vi "WrapStrToFitButtonSize.vi"(0 "String in":string) -> (14 "Wrapped String":string)   [LabVIEW 2017, in "NEVSTOP QD Shortcuts.lvlib"]
uses:
  NEVSTOP QD Shortcuts.lvlib
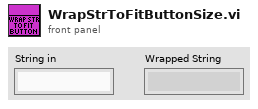
[diagram p1: front panel]
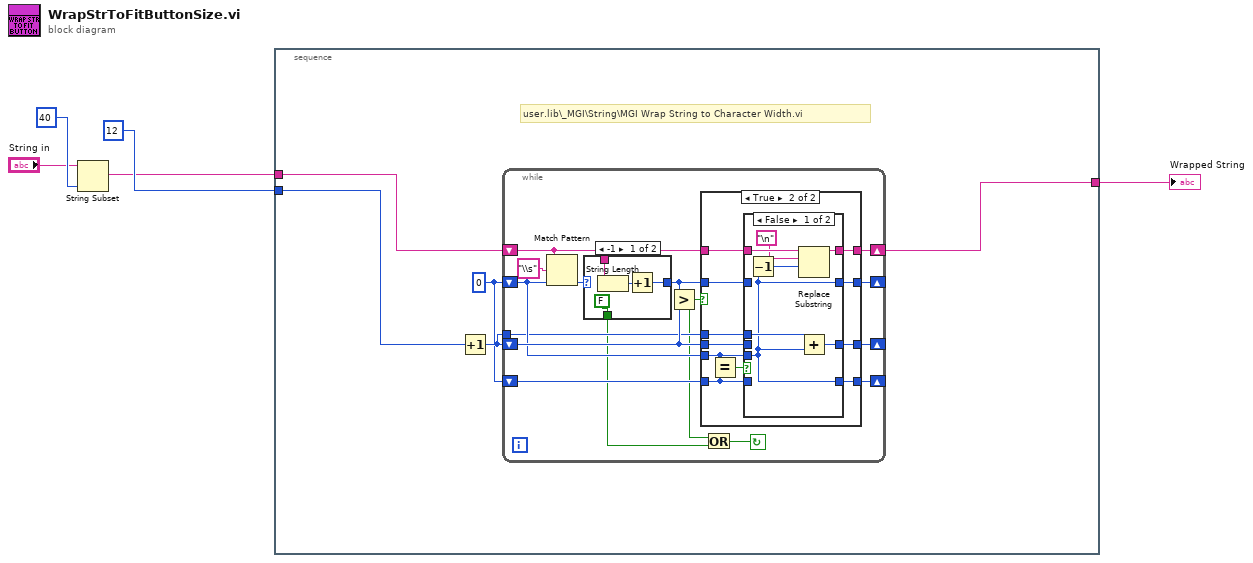
[diagram p0: block diagram]
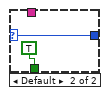
[diagram p2: hidden frame]
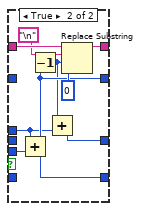
[diagram p4: hidden frame]
diagram:
  n1 = String Subset(string="String in", length (rest)=40 ("length (rest)")) -> (substring=w3:string)  [unwired: 1 in]
  n2 = stacked-sequence {
    tunnel: [w10] -> w2
    tunnel: 12 ("Wrap length(Characters)") -> [w9]
    tunnel: w3 -> [w6]
    frame #0 {
      w7 = 0
      # "user.lib\\_MGI\\String\\MGI Wrap String to Character Width.vi"
      n3 = Increment(x=w9) -> (x+1=w8:i32)
      n4 = while {
        shift-right: [w24] -> w10
        shift-left: w6 -> [w18]
        shift-right: [w23] -> _
        shift-left: w7 -> [w15]
        shift-right: [w21] -> _
        shift-left: w8 -> [w22]
        shift-right: [w16] -> _
        shift-left: w7 -> [w17]
        tunnel: w8 -> [w14]
        stop <- w11 continue-if-true
        n5 = Match Pattern(string=w18, regular expression="\\s", offset (0)=w15) -> (offset past match=w20:i32)  [unwired: 3 out]
        n6 = case shown="-1" w20 {
          selector: w20 -> [_ w31]
          tunnel: [w26 w31] -> w19
          tunnel: w18 -> [w29 _]
          tunnel: [FALSE TRUE] -> w12
          frame -1 {
            n7 = String Length(string=w29) -> (length=w27:i32)
            n8 = Increment(x=w27) -> (x+1=w26:i32)
          }
          frame Default {
          }
        }
        n9 = Greater?(x=w19, y=w22) -> (0:w13:bool)
        n10 = case shown="True" w13 {
          tunnel: w19 -> [w34 w42]
          tunnel: w18 -> [w35 w41]
          tunnel: [w35 w40] -> w24
          tunnel: [w34 w36] -> w23
          tunnel: w22 -> [w33 w43]
          tunnel: [w33 w37] -> w21
          tunnel: w15 -> [_ w45]
          tunnel: w17 -> [w32 w44]
          tunnel: [w32 w39] -> w16
          tunnel: w14 -> [_ w38]
          frame False {
          }
          frame True {
            n11 = Equal?(x=w45, y=w44) -> (x = y?=w46:bool)
            n12 = case shown="False" w46 {
              tunnel: w45 -> [w47 w58]
              tunnel: w44 -> [_ _]
              tunnel: w43 -> [_ _]
              tunnel: w42 -> [_ _]
              tunnel: w41 -> [w53 w62]
              tunnel: [w50 w61] -> w40
              tunnel: [w47 w57] -> w39
              tunnel: w38 -> [w49 w56]
              tunnel: [w48 w54] -> w37
              tunnel: [w47 w57] -> w36
              frame False {
                n13 = Decrement(x=w47) -> (x-1=w52:i32)
                n14 = Replace Substring(3:w52, 4:"\n", 5:w53) -> (1:w50:string)  [unwired: 1 in, 1 out]
                n15 = Add(x=w49, y=w47) -> (x+y=w48:i32)
              }
              frame True {
                n16 = Add(x=w56, y=w58) -> (x+y=w57:i32)
                n17 = Decrement(x=w57) -> (x-1=w55:i32)
                n18 = Add(x=w55, y=w56) -> (x+y=w54:i32)
                n19 = Replace Substring(2:0 ("length (len. of substring)"), 3:w55, 4:"\n", 5:w62) -> (1:w61:string)  [unwired: 1 out]
              }
            }
          }
        }
        n20 = Or(x=w13, y=w12) -> (x .or. y?=w11:bool)
      }
    }
  }
  "Wrapped String" <- w2
